vi "GlobalGetKoherasLaserOnOff.vi"() -> ()   [LabVIEW 2011]
panel:
  out "GetKoherasLaser":bool
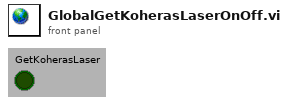
[diagram p1: front panel]
diagram:
